vi "Set Retrieved Items.vi"(8 "error in (no error)":errorcluster, 10 "Retrieved Items":T1[](array[typedef]), 11 "MyItem DAO in":refnum<class "Object DAO.lvclass">) -> (0 "error out":errorcluster, 3 "MyItem DAO out":refnum<class "Object DAO.lvclass">)   [LabVIEW 2020, in "Object DAO.lvclass"]
uses:
  Object DAO.lvclass
  Type Def/Object Information.ctl
  Object DAO.lvclass/Object DAO.ctl
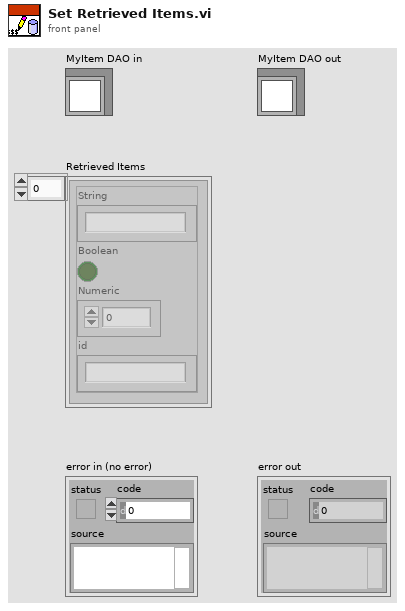
[diagram p1: front panel]
types:
  T1 = typedef "Object DAO.lvclass/Object Information.ctl" = cluster{"String":string, "Boolean":bool, "Numeric":dbl, "id":string}
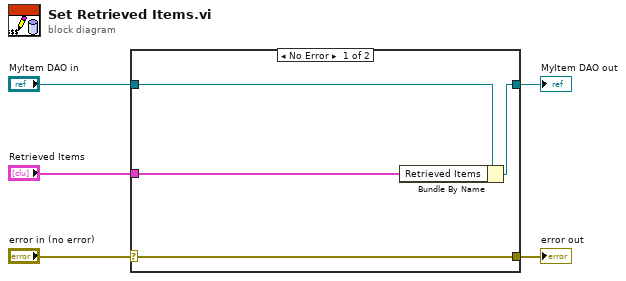
[diagram p0: block diagram]
diagram:
  n1 = case shown="No Error" "error in (no error)" {
    selector: "error in (no error)" -> [w9 w10]
    tunnel: [w9 w10] -> w4
    tunnel: [w7 w11] -> w2
    tunnel: "MyItem DAO in" -> [w8 w11]
    tunnel: "Retrieved Items" -> [w6 _]
    frame No Error {
      n2 = Bundle By Name(cluster=w8, "Retrieved Items"=w6) -> (w7:refnum<class "Object DAO.lvclass">)
    }
    frame Error {
    }
  }
  "error out" <- w4
  "MyItem DAO out" <- w2
